vi "UP-COUNTER-V1.vi"(11 "UPPER LIMIT":dbl=5.0 format="%#_13g") -> (3 "COUNT":dbl)   [LabVIEW 2016]
panel:
  in  "LOWER LIMIT":dbl format="%#_13g"
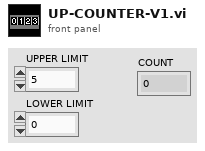
[diagram p1: front panel]
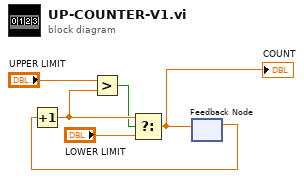
[diagram p0: block diagram]
diagram:
  n1 = feedback #1() -> (w4:dbl)  [unwired: 1 in]
  n2 = Increment(x=w4) -> (x+1=w5:dbl)
  n3 = Greater?(x="UPPER LIMIT", y=w5) -> (0:w2:bool)
  n4 = Select(t=w5, s=w2, f="LOWER LIMIT") -> (s? t:f=w6:dbl)
  "COUNT" <- w6
  n5 = feedback-in #1(w6) -> ()
